vi "Sets the Resistance Value for the dBm Function.vi"(5 "Enable to Query":bool=TRUE, 7 "Enable to Sets":bool=TRUE, 8 "error in":errorcluster, 10 "Resistance Value for dBm":u8(ring) items=["2", "4", "8", "16", "50", "75", "93", "110", "124", "125", "135", "150", "250", "300", "500", "600", "800", "900", "1000", "1200", "8000"], 11 "VISA resource name":refnum<visa-resource-name>) -> (0 "error out":errorcluster, 2 "Return the Resistance Value":string, 3 "VISA resource name out":refnum<visa-resource-name>)   [LabVIEW 2011, in "DMM4.lvlib"]
uses:
  <instrlib>/DMM4/DMM4.lvlib
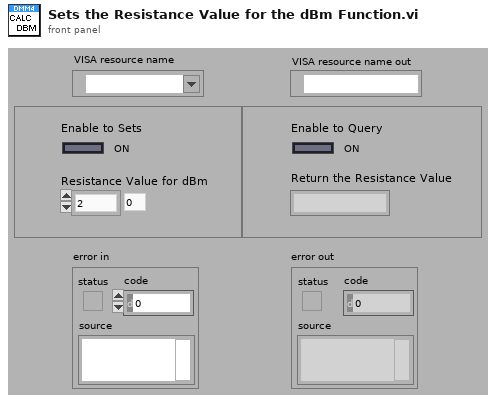
[diagram p1: front panel]
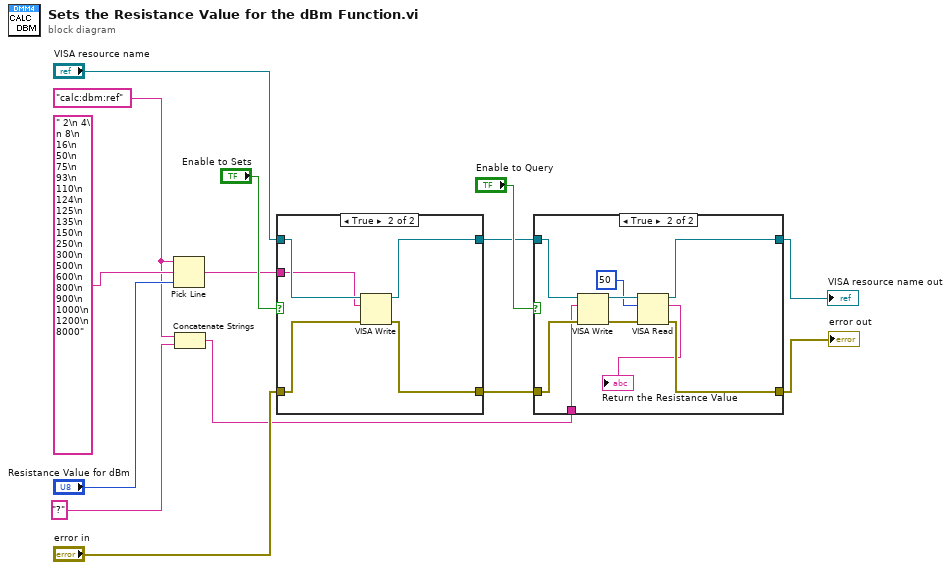
[diagram p0: block diagram]
diagram:
  w11 = "calc:dbm:ref"
  n1 = Pick Line(string ("")=w11, multi-line string=" 2\n 4\n 8\n 16\n 50\n 75\n 93\n 110\n 124\n 125\n 135\n 150\n 250\n 300\n 500\n 600\n 800\n 900\n 1000\n 1200\n 8000", line index="Resistance Value for dBm") -> (output string=w7:string)
  n2 = Concatenate Strings(w11, "?") -> (w1:string)
  n3 = case shown="True" "Enable to Sets" {
    tunnel: "VISA resource name" -> [w16 w21]
    tunnel: "error in" -> [w15 w20]
    tunnel: [w16 w19] -> w5
    tunnel: [w15 w18] -> w4
    tunnel: w7 -> [_ w17]
    frame False {
    }
    frame True {
      n4 = VISA Write(VISA resource name=w21, write buffer=w17, error in (no error)=w20) -> (VISA resource name out=w19:refnum<visa-resource-name>, error out=w18:errorcluster)  [unwired: 1 out]
    }
  }
  n5 = case shown="True" "Enable to Query" {
    tunnel: w5 -> [w23 w29]
    tunnel: w4 -> [w22 w28]
    tunnel: [w23 w27] -> w3
    tunnel: [w22 w26] -> w2
    tunnel: w1 -> [_ w24]
    frame False {
    }
    frame True {
      n6 = VISA Write(VISA resource name=w29, write buffer=w24, error in (no error)=w28) -> (VISA resource name out=w31:refnum<visa-resource-name>, error out=w32:errorcluster)  [unwired: 1 out]
      n7 = VISA Read(VISA resource name=w31, byte count=u32 50, error in (no error)=w32) -> (VISA resource name out=w27:refnum<visa-resource-name>, read buffer=→"Return the Resistance Value":string, error out=w26:errorcluster)  [unwired: 1 out]
    }
  }
  "VISA resource name out" <- w3
  "error out" <- w2
